vi "Organize All Test Data.vi"(8 "error in (no error)":errorcluster, 11 "Test Item PTR From All STDF":refnum<class "PTR.lvclass">[][][](array[class])) -> (0 "error out":errorcluster, 3 "Test Data Out":T1)   [LabVIEW 2018, in "STDF File Parser.lvclass"]
uses:
  STDF File Parser.lvclass
  <userlib>/STDF/PTR/PTR.lvclass
  TestDataMgr/Typedefs/Test Data All.ctl
  TestDataMgr/Typedefs/Test Limits.ctl
  TestDataMgr/Typedefs/Test Raw Data.ctl
  TestDataMgr/TestDataMgr.lvclass
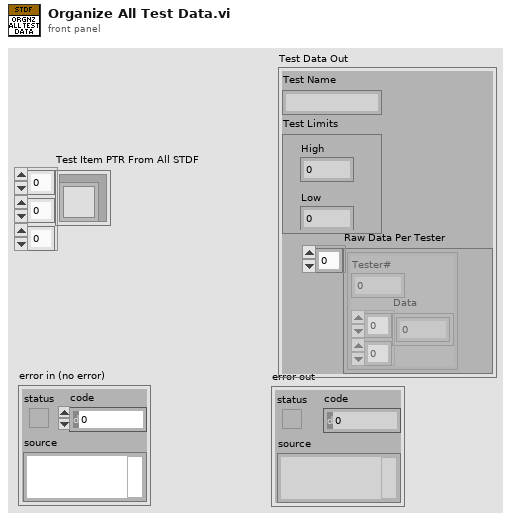
[diagram p1: front panel]
types:
  T1 = typedef "TestDataMgr.lvclass/Test Data All.ctl" = cluster{"Test Name":string, "Test Limits":T2, "Raw Data Per Tester":T3[]}
  T2 = typedef "TestDataMgr.lvclass/Test Limits.ctl" = cluster{"High":dbl, "Low":dbl}
  T3 = typedef "TestDataMgr.lvclass/Test Raw Data.ctl" = cluster{"Data":dbl[][], "Tester#":u8}
  T4 = typedef "STDF File Parser.lvclass/PTR Data.ctl" = cluster{"Result":dbl, "High Limit":dbl, "Low Limit":dbl, "Test Name":string}
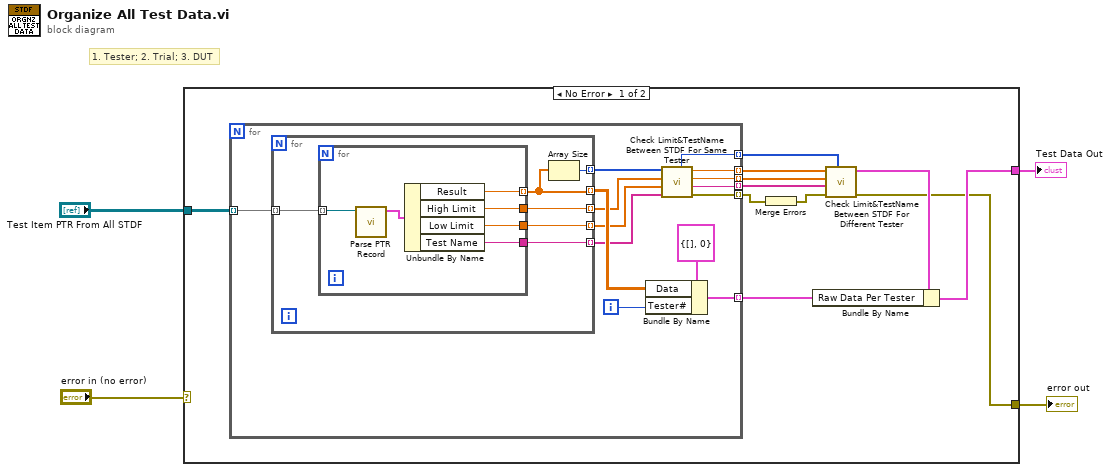
[diagram p0: block diagram]
diagram:
  # "1. Tester; 2. Trial; 3. DUT"
  n1 = case shown="No Error" "error in (no error)" {
    selector: "error in (no error)" -> [_ w42]
    tunnel: [w5 w42] -> w3
    tunnel: "Test Item PTR From All STDF" -> [w15 _]
    tunnel: [w14 _] -> w1
    frame No Error {
      n2 = for {
        tunnel: w15 -> [w29] mode=indexing
        tunnel: [w26] -> w13 mode=indexing
        tunnel: [w20] -> w9 mode=indexing
        tunnel: [w19] -> w8 mode=indexing
        tunnel: [w18] -> w7 mode=indexing
        tunnel: [w17] -> w12 mode=indexing
        tunnel: [w16] -> w10 mode=indexing
        i -> [w27]
        n3 = for {
          tunnel: w29 -> [w35] mode=indexing
          tunnel: [w34] -> w21 mode=indexing
          tunnel: [w33] -> w22 mode=indexing
          tunnel: [w32] -> w23 mode=indexing
          tunnel: [w31] -> w25 mode=indexing
          tunnel: [w30] -> w24 mode=indexing
          n4 = for {
            tunnel: w35 -> [w36] mode=indexing
            tunnel: [w40] -> w34
            tunnel: [w39] -> w33
            tunnel: [w38] -> w32
            tunnel: [w37] -> w31 mode=indexing
            n5 = call "Parse PTR Record.vi"("STDF.lvlib:PTR"=w36) -> ("PTR Data"=w41:T4)  [unwired: 9 in, 1 out]
            n6 = Unbundle By Name(w41) -> ("Result"=w37:dbl, "High Limit"=w38:dbl, "Low Limit"=w39:dbl, "Test Name"=w40:string)
          }
          n7 = Array Size(array=w31) -> (size(s)=w30:i32)
        }
        n8 = Bundle By Name(cluster=T3 {"Data"=[], "Tester#"=0} ("Raw Data Per Tester"), "Data"=w25, "Tester#"=w27) -> (w26:T3)
        n9 = call "Check Limit&TestName Between STDF For Same Tester.vi"("Test Name Array"=w21, "Low Limit Array"=w22, "High Limit Array"=w23, "Result Length Array"=w24) -> ("error out"=w17:errorcluster, "Test Name"=w18:string, "Low Limit"=w19:dbl, "High Limit"=w20:dbl, "Result Length"=w16:i32)  [unwired: 3 in]
      }
      n10 = Merge Errors(w12) -> (w11:errorcluster)
      n11 = call "Check Limit&TestName Between STDF For Different Tester.vi"("Result Length Array"=w10, "error in (no error)"=w11, "Test Name Array"=w7, "Low Limit Array"=w8, "High Limit Array"=w9) -> ("error out"=w5:errorcluster, "Test Data Out"=w6:T1)  [unwired: 5 in]
      n12 = Bundle By Name(cluster=w6, "Raw Data Per Tester"=w13) -> (w14:T1)
    }
    frame Error {
    }
  }
  "error out" <- w3
  "Test Data Out" <- w1
